vi "Update.vi"(8 "error in (no error)":errorcluster, 10 "Message in":refnum<class "UpdateMessage.lvclass">, 11 "AOTF in":refnum<class "AOTF.lvclass">) -> (0 "error out":errorcluster, 3 "AOTF out":refnum<class "AOTF.lvclass">)   [LabVIEW 2012, in "AOTF.lvclass"]
doc: "The update method processes the command 'update'. \n\nThe command 'update' is used for receiving new values to be set to the private data of the class. This could be seen as a public set method for setting new parameters to the private class data."
uses:
  AOTF.lvclass
  <vilib>/Distrio/Murmex/UpdateMessage/UpdateMessage.lvclass
  AOTF.lvclass/AOTF.ctl
  Controls/laser line ring.ctl
  Controls/Illumination arm.ctl
  <vilib>/Distrio/Murmex/Murmex/Murmex.lvclass
panel:
  # "This method is called when the UPDATE\ntrigger is sent. \n\nOverride this method when your component needs to\nrespond to this trigger. \n\nCall parent for proper implementation"
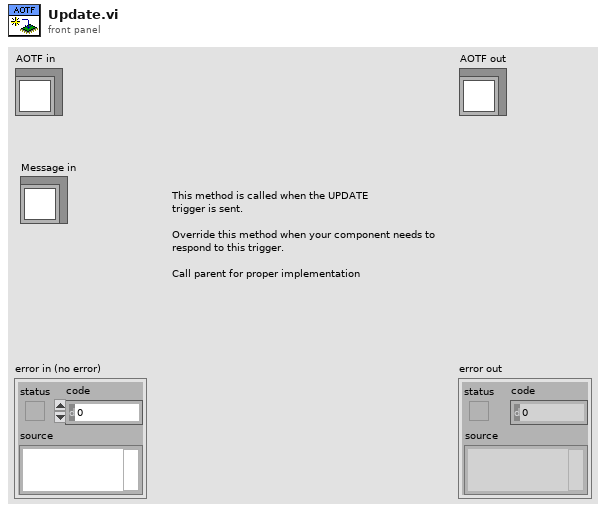
[diagram p1: front panel]
types:
  T1 = typedef "AOTF.lvclass/Illumination arm.ctl" = enum16{"Florence", "Prato"}
  T2 = typedef "AOTF.lvclass/laser line ring.ctl" = u8
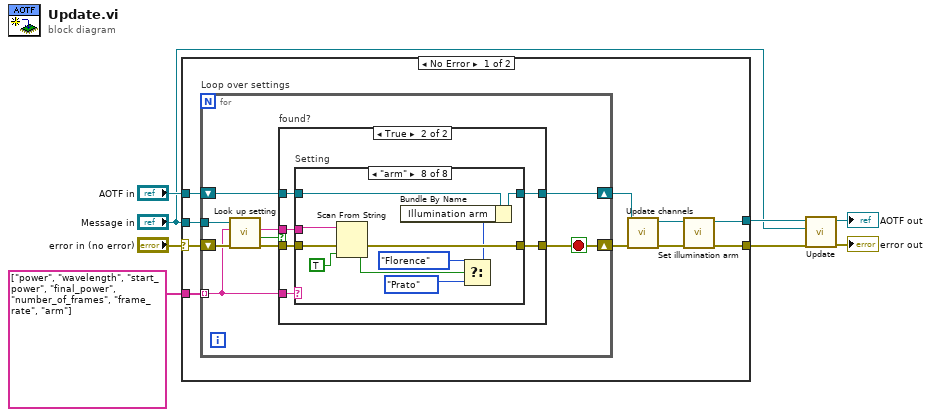
[diagram p0: block diagram]
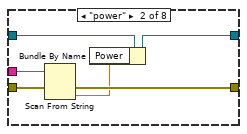
[diagram p4: hidden frame]
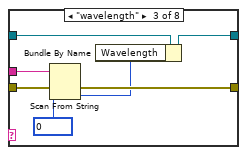
[diagram p5: hidden frame]
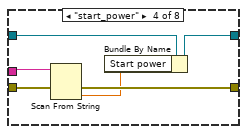
[diagram p6: hidden frame]
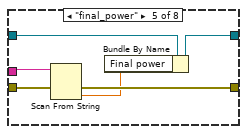
[diagram p7: hidden frame]
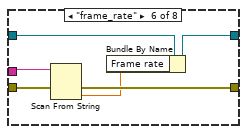
[diagram p8: hidden frame]
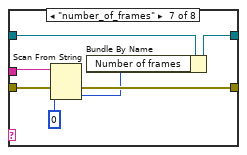
[diagram p9: hidden frame]
diagram:
  n1 = case shown="No Error" "error in (no error)" {
    selector: "error in (no error)" -> [w18 w86]
    tunnel: string[] ["power", "wavelength", "start_power", "final_power", "number_of_frames", "frame_rate", "arm"] ("key chains") -> [w17 _]
    tunnel: "Message in" -> [w16 _]
    tunnel: "AOTF in" -> [w15 w87]
    tunnel: [w9 w86] -> w3
    tunnel: [w11 w87] -> w2
    frame No Error {
      n2 = for "Loop over settings" {
        shift-right: [w21] -> w13
        shift-left: w18 -> [w27]
        tunnel: w17 -> [w22] mode=indexing
        tunnel: w16 -> [w26]
        shift-right: [w19] -> w14
        shift-left: w15 -> [w20]
        stop <- w21 stop-if-true
        n3 = call <vilib>:"Look up setting.vi"("error in (no error)"=w27, "tag name"=w22, "UpdateMessage in"=w26) -> ("error out"=w23:errorcluster, "found?"=w25:bool, "value"=w24:string)  [unwired: 5 in, 1 out]
        n4 = case "found?" shown="True" w25 {
          tunnel: w24 -> [_ w34]
          tunnel: w23 -> [w29 w33]
          tunnel: w22 -> [_ w35]
          tunnel: [w29 w32] -> w21
          tunnel: w20 -> [w28 w31]
          tunnel: [w28 w30] -> w19
          frame False {
          }
          frame True {
            n5 = case "Setting" shown="\"arm\"" w35 {
              tunnel: w34 -> [_ w41 w49 w54 w60 w66 w73 w83]
              tunnel: w33 -> [w37 w40 w50 w56 w62 w68 w75 w85]
              tunnel: [w37 w39 w46 w55 w61 w67 w74 w84] -> w32
              tunnel: w31 -> [w36 w43 w48 w53 w59 w65 w72 w82]
              tunnel: [w36 w42 w47 w52 w58 w64 w71 w81] -> w30
              frame Default {
              }
              frame "power" {
                n6 = Scan From String(input string=w41, error in=w40) -> (error out=w39:errorcluster, output 1=w38:dbl)  [unwired: 3 in, 2 out]
                n7 = Bundle By Name(cluster=w43, "Power"=w38) -> (w42:refnum<class "AOTF.lvclass">)
              }
              frame "wavelength" {
                w44 = T2 0 items=["405nm"=1, "445nm"=5, "491nm"=2, "515nm"=3, "561nm"=4] ("Settings cluster.Wavelength")
                n8 = Scan From String(input string=w49, error in=w50, default 1=w44) -> (error out=w46:errorcluster, output 1=w45:T2)  [unwired: 2 in, 2 out]
                n9 = Bundle By Name(cluster=w48, "Wavelength"=w45) -> (w47:refnum<class "AOTF.lvclass">)
              }
              frame "start_power" {
                n10 = Scan From String(input string=w54, error in=w56) -> (error out=w55:errorcluster, output 1=w51:dbl)  [unwired: 3 in, 2 out]
                n11 = Bundle By Name(cluster=w53, "Start power"=w51) -> (w52:refnum<class "AOTF.lvclass">)
              }
              frame "final_power" {
                n12 = Scan From String(input string=w60, error in=w62) -> (error out=w61:errorcluster, output 1=w57:dbl)  [unwired: 3 in, 2 out]
                n13 = Bundle By Name(cluster=w59, "Final power"=w57) -> (w58:refnum<class "AOTF.lvclass">)
              }
              frame "frame_rate" {
                n14 = Scan From String(input string=w66, error in=w68) -> (error out=w67:errorcluster, output 1=w63:dbl)  [unwired: 3 in, 2 out]
                n15 = Bundle By Name(cluster=w65, "Frame rate"=w63) -> (w64:refnum<class "AOTF.lvclass">)
              }
              frame "number_of_frames" {
                n16 = Scan From String(input string=w73, error in=w75, default 1=0 ("Settings cluster.Number of frames")) -> (error out=w74:errorcluster, output 1=w70:i32)  [unwired: 2 in, 2 out]
                n17 = Bundle By Name(cluster=w72, "Number of frames"=w70) -> (w71:refnum<class "AOTF.lvclass">)
              }
              frame "arm" {
                n18 = Scan From String(input string=w83, error in=w85, default 1=TRUE) -> (error out=w84:errorcluster, output 1=w79:bool)  [unwired: 2 in, 2 out]
                n19 = Select(t=Illumination_arm."Florence" ("Settings cluster.Illumination arm"), s=w79, f=Illumination_arm."Prato" ("Settings cluster.Illumination arm")) -> (s? t:f=w76:T1)
                n20 = Bundle By Name(cluster=w82, "Illumination arm"=w76) -> (w81:refnum<class "AOTF.lvclass">)
              }
            }
          }
        }
      }
      n21 = call-dynamic "Update channels.vi"("error in (no error)"=w13, "AOTF in"=w14) -> ("error out"=w10:errorcluster, "AOTF out"=w12:refnum<class "AOTF.lvclass">)  [unwired: 8 in]
      n22 = call-dynamic "Set illumination arm.vi"("error in (no error)"=w10, "AOTF in"=w12) -> ("error out"=w9:errorcluster, "AOTF out"=w11:refnum<class "AOTF.lvclass">)  [unwired: 8 in]
    }
    frame Error {
    }
  }
  n23 = call-parent "Update.vi"("error in (no error)"=w3, "Message in"="Message in", "Murmex in"=w2) -> ("error out"=→"error out":errorcluster, "Murmex out"=→"AOTF out":refnum<class "AOTF.lvclass">)  [unwired: 7 in]
